vi "Read Tim Obs.vi"(8 "error in":errorcluster, 11 "tCRD in":refnum<class "Aircraft OPCCRD.lvclass">) -> (0 "error out":errorcluster, 2 "Tim Obs":refnum<class "Tim File Observer.lvclass">, 3 "tCRD out":refnum<class "Aircraft OPCCRD.lvclass">)   [LabVIEW 2015, in "Aircraft OPCCRD.lvclass"]
uses:
  Aircraft OPCCRD.lvclass
  File Observer/Tim File Observer.lvclass
  Aircraft OPCCRD.lvclass/Aircraft OPCCRD.ctl
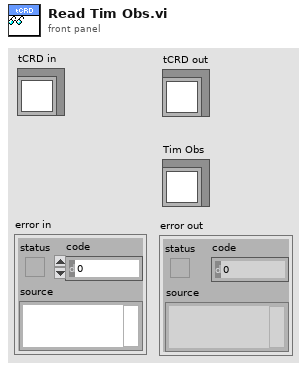
[diagram p1: front panel]
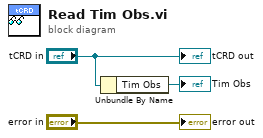
[diagram p0: block diagram]
diagram:
  n1 = Unbundle By Name("tCRD in") -> ("Tim Obs"=→"Tim Obs":refnum<class "Tim File Observer.lvclass">)
  "error out" <- "error in"
  "tCRD out" <- "tCRD in"
